vi "Limit PWM Value.vi"(11 "PWM In":dbl) -> (3 "PWM Out":dbl)   [LabVIEW 2018]
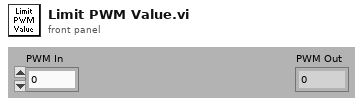
[diagram p1: front panel]
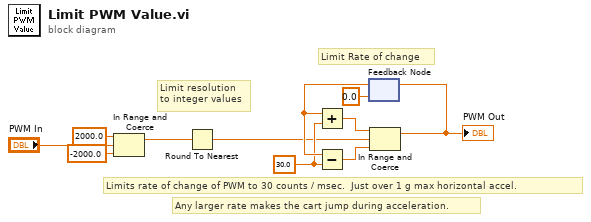
[diagram p0: block diagram]
diagram:
  w4 = 30.0 ("y")
  # "Any larger rate makes the cart jump during acceleration."
  # "Limits rate of change of PWM to 30 counts / msec.  Just over 1 g max horizontal accel."
  # "Limit resolution\nto integer values"
  # "Limit Rate of change"
  n1 = In Range and Coerce(upper limit=2000.0, x="PWM In", lower limit=-2000.0) -> (coerced(x)=w8:dbl)  [unwired: 1 out]
  n2 = Round To Nearest(number=w8) -> (nearest integer value=w3:dbl)
  n3 = feedback #1(0.0) -> (w6:dbl)
  n4 = Add(x=w6, y=w4) -> (x+y=w7:dbl)
  n5 = Subtract(x=w6, y=w4) -> (x-y=w5:dbl)
  n6 = In Range and Coerce(upper limit=w7, x=w3, lower limit=w5) -> (coerced(x)=w2:dbl)  [unwired: 1 out]
  "PWM Out" <- w2
  n7 = feedback-in #1(w2) -> ()
